vi "numAndTempStats.vi"(8 "Stat. Limits":cluster{"Start Index":i32, "Length":i32}, 9 "Stats Flag":bool, 11 "strip chart properties":T1) -> (3 "Num and Temp Stats":T2 {"Std. Y Temp" format="%#_3p"; "Mean Y Temp" format="%#_3p"; "Mean X Temp" format="%#_3p"; "Mean Num." format="%#_3p"; "Std. X Temp" format="%#_3p"; "Std. Num" format="%#_3p"})   [LabVIEW 2016]
uses:
  Controls/numAndTempStats.ctl
  <vilib>/Analysis/NI_AALBase.lvlib
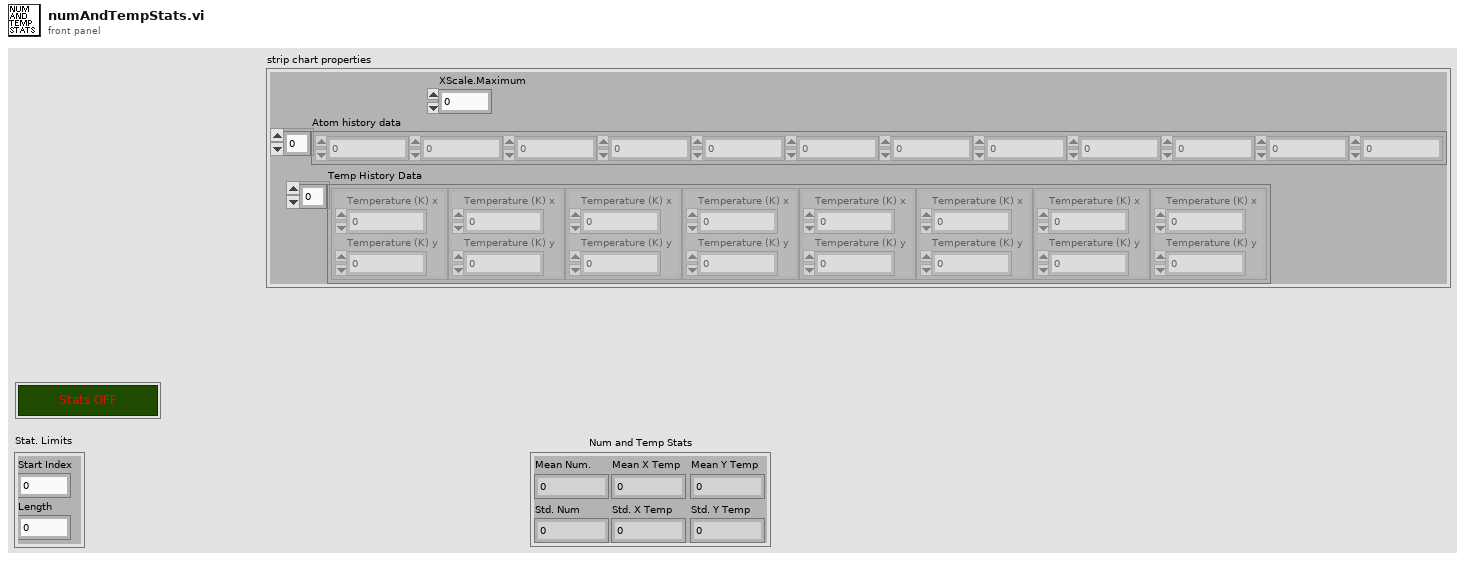
[diagram p1: front panel]
types:
  T1 = cluster{"XScale.Maximum":dbl, "Atom history data":dbl[], "Temp History Data":cluster{"Temperature (K) x":dbl, "Temperature (K) y":dbl}[]}
  T2 = typedef "numAndTempStats.ctl" = cluster{"Mean Num.":dbl, "Std. Num":dbl, "Mean X Temp":dbl, "Std. X Temp":dbl, "Mean Y Temp":dbl, "Std. Y Temp":dbl}
  T3 = cluster{"Temperature (K) x":dbl, "Temperature (K) y":dbl}[]
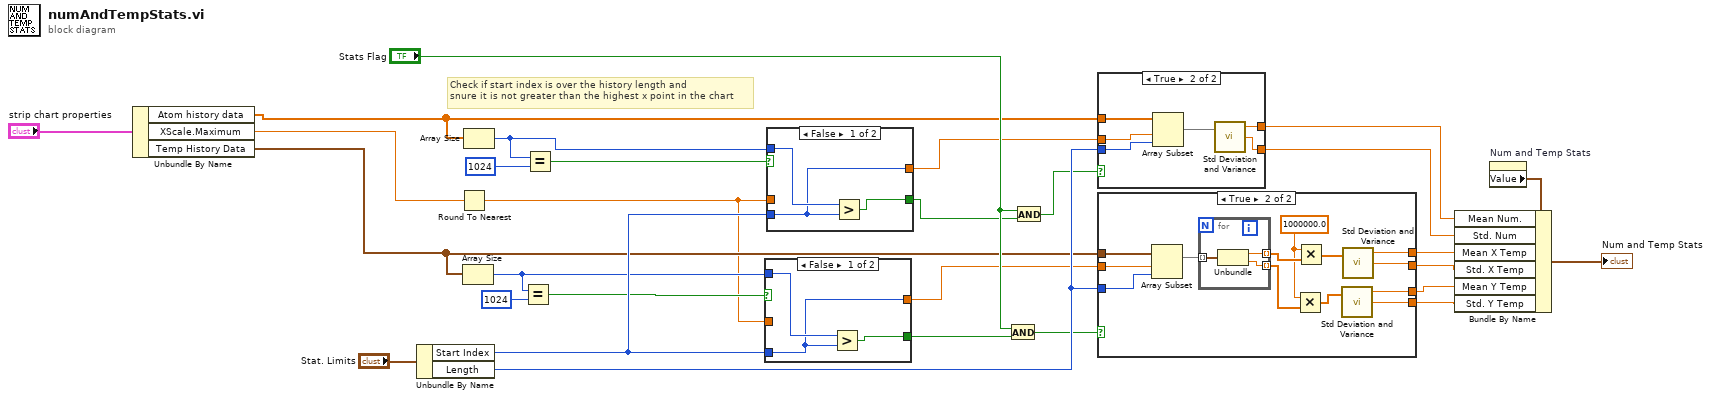
[diagram p0: block diagram]
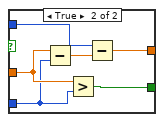
[diagram p2: hidden frame]
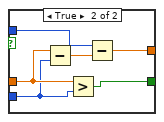
[diagram p3: hidden frame]
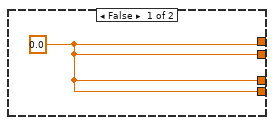
[diagram p4: hidden frame]
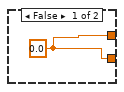
[diagram p5: hidden frame]
diagram:
  # "Check if start index is over the history length and \nsnure it is not greater than the highest x point in the chart"
  n1 = Unbundle By Name("strip chart properties") -> ("Atom history data"=w6:dbl[], "XScale.Maximum"=w5:dbl, "Temp History Data"=w4:T3)
  n2 = Unbundle By Name("Stat. Limits") -> ("Start Index"=w10:i32, "Length"=w21:i32)
  n3 = Round To Nearest(number=w5) -> (nearest integer value=w2:dbl)
  n4 = Array Size(array=w4) -> (size(s)=w8:i32)
  n5 = Array Size(array=w6) -> (size(s)=w12:i32)
  n6 = Equal?(x=w8, y=1024) -> (x = y?=w7:bool)
  n7 = Equal?(x=w12, y=1024) -> (x = y?=w13:bool)
  n8 = case shown="False" w7 {
    tunnel: [w30 w38] -> w1
    tunnel: w10 -> [w30 w34]
    tunnel: w2 -> [_ w35]
    tunnel: [w32 w33] -> w11
    tunnel: w8 -> [w31 w36]
    frame False {
      n9 = Greater?(x=w31, y=w30) -> (0:w32:bool)
    }
    frame True {
      n10 = Subtract(x=w35, y=w34) -> (x-y=w37:dbl)
      n11 = Greater?(x=w35, y=w34) -> (0:w33:bool)
      n12 = Subtract(x=w36, y=w37) -> (x-y=w38:dbl)
    }
  }
  n13 = case shown="False" w13 {
    tunnel: [w39 w47] -> w16
    tunnel: w10 -> [w39 w43]
    tunnel: w2 -> [_ w44]
    tunnel: [w41 w42] -> w15
    tunnel: w12 -> [w40 w45]
    frame False {
      n14 = Greater?(x=w40, y=w39) -> (0:w41:bool)
    }
    frame True {
      n15 = Subtract(x=w44, y=w43) -> (x-y=w46:dbl)
      n16 = Greater?(x=w44, y=w43) -> (0:w42:bool)
      n17 = Subtract(x=w45, y=w46) -> (x-y=w47:dbl)
    }
  }
  n18 = And(x="Stats Flag", y=w11) -> (x .and. y?=w19:bool)
  n19 = And(x="Stats Flag", y=w15) -> (x .and. y?=w18:bool)
  n20 = case shown="True" w18 {
    tunnel: w16 -> [_ w53]
    tunnel: w21 -> [_ w52]
    tunnel: w6 -> [_ w54]
    tunnel: [w48 w51] -> w27
    tunnel: [w48 w50] -> w28
    frame False {
      w48 = 0.0
    }
    frame True {
      n21 = Array Subset(array=w54, index=w53, length=w52) -> (w49:dbl[])
      n22 = call <vilib>:"Std Deviation and Variance.vi"("X"=w49) -> ("mean"=w51:dbl, "standard deviation"=w50:dbl)  [unwired: 1 in, 1 out]
    }
  }
  n23 = case shown="True" w19 {
    tunnel: [w55 w68] -> w23
    tunnel: [w55 w67] -> w24
    tunnel: w21 -> [_ w65]
    tunnel: w4 -> [_ w66]
    tunnel: [w55 w63] -> w25
    tunnel: [w55 w62] -> w26
    tunnel: w1 -> [_ w56]
    frame False {
      w55 = 0.0
    }
    frame True {
      w57 = 1000000.0 ("x")
      n24 = Array Subset(array=w66, index=w56, length=w65) -> (w64:T3)
      n25 = for {
        tunnel: w64 -> [w71] mode=indexing
        tunnel: [w70] -> w59 mode=indexing
        tunnel: [w69] -> w58 mode=indexing
        n26 = Unbundle(w71) -> ("Temperature (K) x"=w70:dbl, "Temperature (K) y"=w69:dbl)
      }
      n27 = Multiply(x=w57, y=w58) -> (x*y=w61:dbl[])
      n28 = Multiply(x=w57, y=w59) -> (x*y=w60:dbl[])
      n29 = call <vilib>:"Std Deviation and Variance.vi"("X"=w61) -> ("mean"=w63:dbl, "standard deviation"=w62:dbl)  [unwired: 1 in, 1 out]
      n30 = call <vilib>:"Std Deviation and Variance.vi"("X"=w60) -> ("mean"=w68:dbl, "standard deviation"=w67:dbl)  [unwired: 1 in, 1 out]
    }
  }
  n31 = property on="Num and Temp Stats" class="Clust (strict)"() -> ("Value"=w22:T2)  [unwired: 2 in, 2 out]
  n32 = Bundle By Name(cluster=w22, "Mean Num."=w27, "Std. Num"=w28, "Mean X Temp"=w23, "Std. X Temp"=w24, "Mean Y Temp"=w25, "Std. Y Temp"=w26) -> (→"Num and Temp Stats":T2)
